vi "Service Location FGV.vi"(8 "error in":errorcluster, 9 "location unique id in":u64, 10 "resolve service request":T2, 11 "action":T1) -> (0 "error out":errorcluster, 1 "location unique id out":u64, 3 "service location":T3)   [LabVIEW 2020, in "MeasurementLink Discovery.lvlib"]
uses:
  MeasurementLink Discovery.lvlib
  MeasurementLink Discovery Client/RPC Messages/ni_measurementlink_discovery_v1_ServiceLocation.ctl
  MeasurementLink Discovery Client/RPC Messages/ni_measurementlink_discovery_v1_ResolveServiceRequest.ctl
  Service Location FGV Action.ctl
  MeasurementLink gRPC Utilities/TypeDefs/Service Location Value.ctl
  <vilib>/Utility/miscctls.llb/LVMapReplaceAction.ctl
  MeasurementLink Discovery Client/MeasurementLink Discovery Client.lvlib
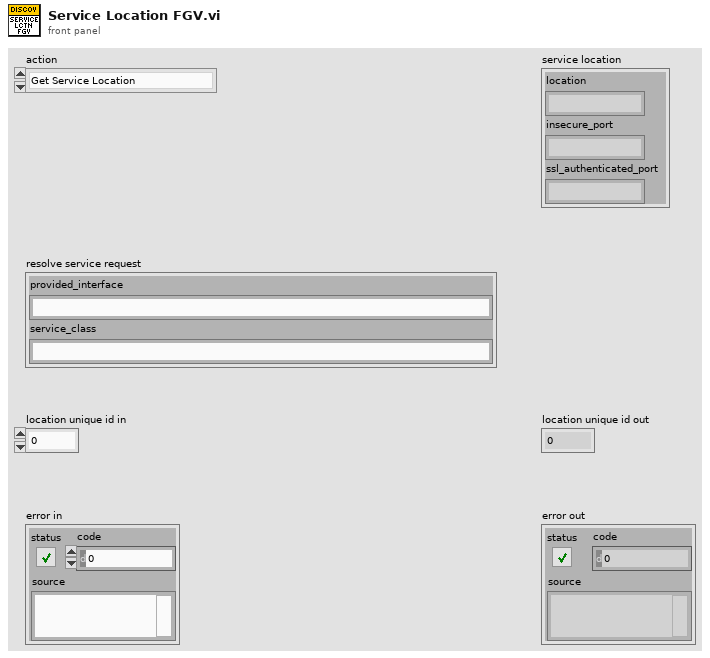
[diagram p1: front panel]
types:
  T1 = typedef "MeasurementLink Discovery.lvlib/Service Location FGV Action.ctl" = enum16{"Get Service Location", "Reresolve Service Location"}
  T2 = typedef "MeasurementLink Discovery Client.lvlib/ni_measurementlink_discovery_v1_ResolveServiceRequest.ctl" = cluster{"provided_interface":string, "service_class":string}
  T3 = typedef "MeasurementLink Discovery Client.lvlib/ni_measurementlink_discovery_v1_ServiceLocation.ctl" = cluster{"location":string, "insecure_port":string, "ssl_authenticated_port":string}
  T4 = typedef "MeasurementLink Discovery.lvlib/Service Location Value.ctl" = cluster{"response data":T3, "unique id":u64}
  T5 = typedef "LVMapReplaceAction.ctl" = enum32{"Modify Entry only if found", "Add or Modify Entry", "Delete Entry"}
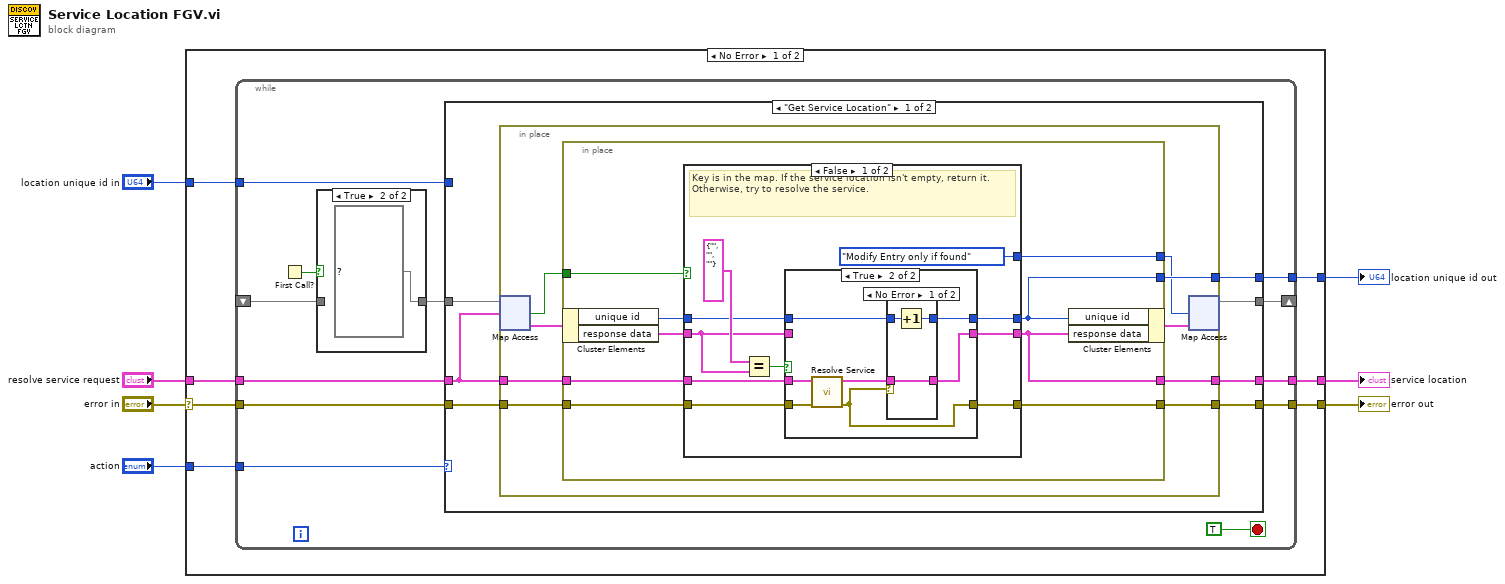
[diagram p0: block diagram]
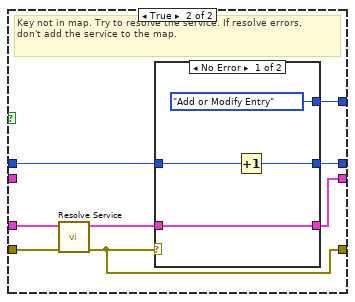
[diagram p5: hidden frame]
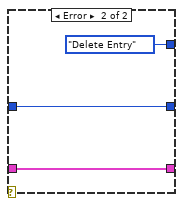
[diagram p6: hidden frame]
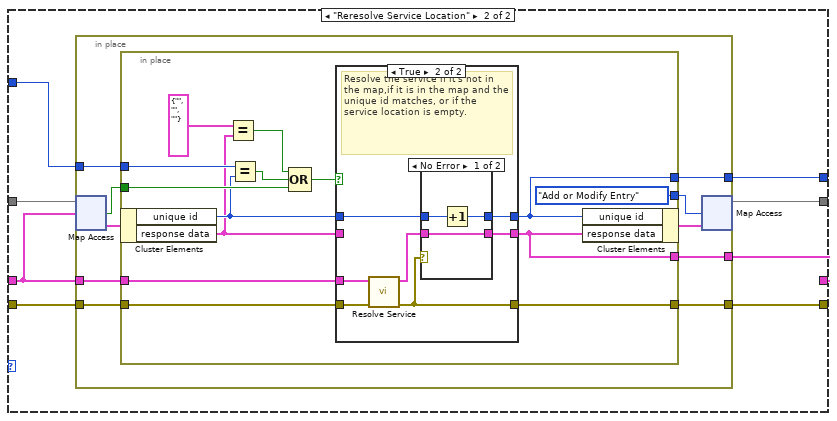
[diagram p7: hidden frame]
diagram:
  n1 = case shown="No Error" "error in" {
    selector: "error in" -> [w14 w139]
    tunnel: [w11 w139] -> w5
    tunnel: [w13 _] -> w7
    tunnel: "resolve service request" -> [w12 _]
    tunnel: "action" -> [w10 _]
    tunnel: [w9 _] -> w2
    tunnel: "location unique id in" -> [w8 _]
    frame No Error {
      n2 = while {
        shift-right: [w23] -> _
        shift-left: _ -> [w20]
        tunnel: w14 -> [w18]
        tunnel: [w25] -> w13
        tunnel: w12 -> [w24]
        tunnel: [w22] -> w11
        tunnel: w10 -> [w21]
        tunnel: [w16] -> w9
        tunnel: w8 -> [w15]
        stop <- TRUE stop-if-true
        n3 = First Call?() -> (First Call?: T/F=w17:bool)
        n4 = case shown="True" w17 {
          tunnel: w20 -> [w27 _]
          tunnel: [w27 map{T2, T4} {} ("map")] -> w19
          frame False {
          }
          frame True {
          }
        }
        n5 = case shown="\"Get Service Location\"" w21 {
          tunnel: w19 -> [w32 w100]
          tunnel: [w35 w94] -> w25
          tunnel: w24 -> [w30 w98]
          tunnel: w18 -> [w33 w97]
          tunnel: [w31 w95] -> w23
          tunnel: [w34 w96] -> w22
          tunnel: [w29 w93] -> w16
          tunnel: w15 -> [_ w99]
          frame "Get Service Location" {
            n6 = in-place {
              in-place-border: w33 -> [w44]
              in-place-border: [w39] -> w35
              in-place-border: [w43] -> w34
              in-place-border: w30 -> [w41]
              in-place-border: [w40] -> w29
              n7 = in-place-map #1(w32, w30) -> (w38:T4, w42:bool)  [unwired: 1 in]
              n8 = in-place {
                in-place-border: w44 -> [w53]
                in-place-border: [w52] -> w43
                in-place-border: w42 -> [w45]
                in-place-border: w41 -> [w51]
                in-place-border: [w49] -> w40
                in-place-border: [w48] -> w39
                in-place-border: [w47] -> w36
                n9 = in-place-cluster #2(w38) -> ("unique id"=w50:u64, "response data"=w46:T3)
                n10 = case shown="False" w45 {
                  tunnel: w53 -> [w60 w85]
                  tunnel: [w59 w83] -> w52
                  tunnel: w51 -> [w57 w84]
                  tunnel: w50 -> [w56 w82]
                  tunnel: [w55 w81] -> w49
                  tunnel: w46 -> [w54 _]
                  tunnel: [w58 w79] -> w48
                  tunnel: [LVMapReplaceAction."Modify Entry only if found" ("action") w78] -> w47
                  frame False {
                    # "Key is in the map. If the service location isn't empty, return it. Otherwise, try to resolve the service."
                    n11 = Equal?(x=T3 {"location"="", "insecure_port"="", "ssl_authenticated_port"=""} ("y"), y=w54) -> (x = y?=w61:bool)
                    n12 = case shown="True" w61 {
                      tunnel: w60 -> [w66 w73]
                      tunnel: [w66 w71] -> w59
                      tunnel: [w64 w69] -> w58
                      tunnel: w57 -> [_ w72]
                      tunnel: w56 -> [w65 w68]
                      tunnel: [w65 w67] -> w55
                      tunnel: w54 -> [w64 _]
                      frame False {
                      }
                      frame True {
                        n13 = call "Resolve Service.vi"("error in"=w73, "request data"=w72) -> ("error out"=w71:errorcluster, "response data"=w70:T3)  [unwired: 8 in]
                        n14 = case shown="No Error" w71 {
                          tunnel: w70 -> [w76 _]
                          tunnel: [w76 _] -> w69
                          tunnel: w68 -> [w75 w77]
                          tunnel: [w74 w77] -> w67
                          frame No Error {
                            n15 = Increment(x=w75) -> (x+1=w74:u64)
                          }
                          frame Error {
                          }
                        }
                      }
                    }
                  }
                  frame True {
                    # "Key not in map. Try to resolve the service. If resolve errors,\ndon't add the service to the map."
                    n16 = call "Resolve Service.vi"("error in"=w85, "request data"=w84) -> ("error out"=w83:errorcluster, "response data"=w80:T3)  [unwired: 8 in]
                    n17 = case shown="No Error" w83 {
                      tunnel: w82 -> [w89 w92]
                      tunnel: [w88 w92] -> w81
                      tunnel: w80 -> [w87 w90]
                      tunnel: [w87 w90] -> w79
                      tunnel: [LVMapReplaceAction."Add or Modify Entry" ("action") LVMapReplaceAction."Delete Entry" ("action")] -> w78
                      frame No Error {
                        n18 = Increment(x=w89) -> (x+1=w88:u64)
                      }
                      frame Error {
                      }
                    }
                  }
                }
                n19 = in-place-cluster #2("unique id"=w49, "response data"=w48) -> (w37:T4)
              }
              n20 = in-place-map #1(w37, w36) -> (w31:map{T2, T4})  [unwired: 2 out]
            }
          }
          frame "Reresolve Service Location" {
            n21 = in-place {
              in-place-border: w99 -> [w110]
              in-place-border: w98 -> [w108]
              in-place-border: w97 -> [w107]
              in-place-border: [w106] -> w96
              in-place-border: [w103] -> w94
              in-place-border: [w102] -> w93
              n22 = in-place-map #3(w100, w98) -> (w105:T4, w109:bool)  [unwired: 1 in]
              n23 = in-place {
                in-place-border: w110 -> [w124]
                in-place-border: w109 -> [w118]
                in-place-border: w108 -> [w121]
                in-place-border: w107 -> [w120]
                in-place-border: [w119] -> w106
                in-place-border: [w117] -> w103
                in-place-border: [w115] -> w102
                in-place-border: [LVMapReplaceAction."Add or Modify Entry" ("action")] -> w101
                n24 = in-place-cluster #4(w105) -> ("unique id"=w116:u64, "response data"=w113:T3)
                n25 = Equal?(x=T3 {"location"="", "insecure_port"="", "ssl_authenticated_port"=""} ("y"), y=w113) -> (x = y?=w111:bool)
                n26 = Equal?(x=w124, y=w116) -> (x = y?=w122:bool)
                n27 = Compound Arithmetic op=OR(w111, w122, w118) -> (w123:bool)
                n28 = case shown="True" w123 {
                  tunnel: w121 -> [_ w134]
                  tunnel: w120 -> [w127 w133]
                  tunnel: [w127 w132] -> w119
                  tunnel: [w125 w130] -> w117
                  tunnel: w116 -> [w126 w129]
                  tunnel: [w126 w128] -> w115
                  tunnel: w113 -> [w125 _]
                  frame False {
                    # "The key is in the map and the unique id doesn't match, which means the service was already re-resolved."
                  }
                  frame True {
                    # "Resolve the service if it's not in the map,if it is in the map and the unique id matches, or if the service location is empty."
                    n29 = call "Resolve Service.vi"("error in"=w133, "request data"=w134) -> ("error out"=w132:errorcluster, "response data"=w131:T3)  [unwired: 8 in]
                    n30 = case shown="No Error" w132 {
                      tunnel: w131 -> [w137 _]
                      tunnel: [w137 _] -> w130
                      tunnel: w129 -> [w136 w138]
                      tunnel: [w135 w138] -> w128
                      frame No Error {
                        n31 = Increment(x=w136) -> (x+1=w135:u64)
                      }
                      frame Error {
                      }
                    }
                  }
                }
                n32 = in-place-cluster #4("unique id"=w115, "response data"=w117) -> (w104:T4)
              }
              n33 = in-place-map #3(w104, w101) -> (w95:map{T2, T4})  [unwired: 2 out]
            }
          }
        }
      }
    }
    frame Error {
    }
  }
  "service location" <- w7
  "error out" <- w5
  "location unique id out" <- w2
